vi "test Add Import Deploy.vi"(8 "error in":errorcluster, 11 "TestCase in":refnum<class "Examples.lvclass">) -> (0 "error out":errorcluster, 3 "TestCase out":refnum<class "Examples.lvclass">)   [LabVIEW 2024, in "Examples.lvclass"]
uses:
  Examples.lvclass
  C:/Program Files/National Instruments/LabVIEW 2024/vi.lib/NI/VeriStand Custom Device Testing Tools/VeriStandTestCase/VeriStandTestCase.lvclass
  Examples.lvclass/Examples.ctl
  7f6914e5-79d7-41a5-a6cd-be6651e4326d.vi
  <vilib>/addons/_JKI Toolkits/VI Tester/TestCase.llb/TestCase.lvclass
  C:/Program Files/National Instruments/LabVIEW 2024/vi.lib/addons/_JKI Toolkits/VI Tester/TestCase.llb/TestCase.lvclass
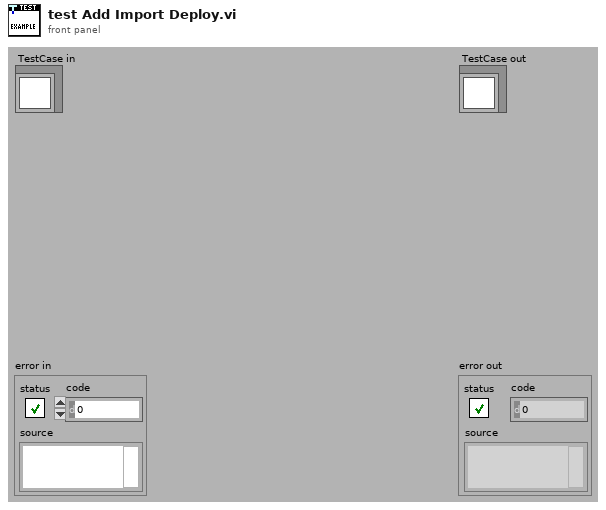
[diagram p1: front panel]
types:
  T1 = typedef "NI_VS Workspace ExecutionAPI.lvlib/WorkspaceAPI.ctl" = refnum<k24>
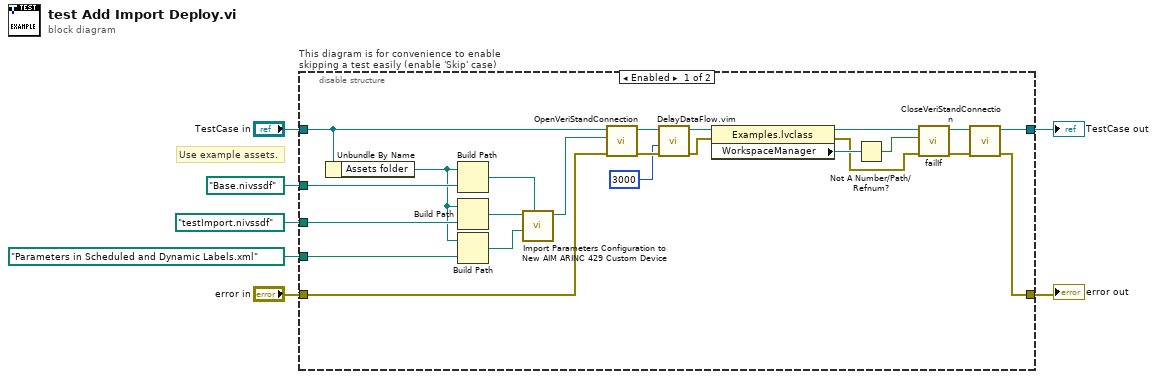
[diagram p0: block diagram]
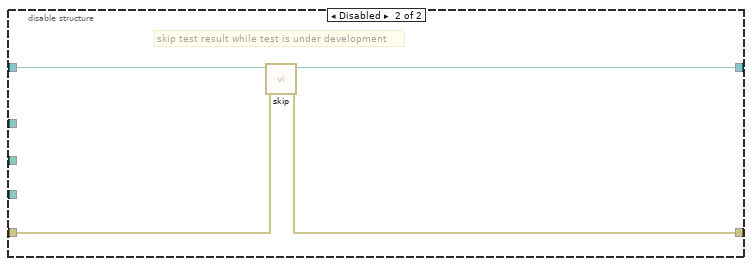
[diagram p2: hidden frame]
diagram:
  # "Use example assets."
  n1 = disable-structure "This diagram is for convenience to enable skipping a test easily (enable 'Skip' case)" shown="Enabled" {
    disable-tunnel: "TestCase in" -> [w16 w33]
    disable-tunnel: [w17 w31] -> w4
    disable-tunnel: [w18 w32] -> w6
    disable-tunnel: "error in" -> [w15 w30]
    disable-tunnel: path "Parameters in Scheduled and Dynamic Labels.xml" ("name or relative path") -> [w29 _]
    disable-tunnel: path "Base.nivssdf" ("name or relative path") -> [w13 _]
    disable-tunnel: path "testImport.nivssdf" ("name or relative path") -> [w12 _]
    frame Enabled {
      n2 = Unbundle By Name(w16) -> ("Assets folder"=w11:path)
      n3 = Build Path(base path=w11, name or relative path=w13) -> (appended path=w8:path)
      n4 = Build Path(base path=w11, name or relative path=w12) -> (appended path=w9:path)
      n5 = Build Path(base path=w11, name or relative path=w29) -> (appended path=w10:path)
      n6 = call "Import Parameters Configuration to New AIM ARINC 429 Custom Device.vi"("Base System Definition File"=w8, "Parameters Configuration File"=w10, "Output System Definition File"=w9) -> ("AIM ARINC 429 System Definition"=w14:path)  [unwired: 8 in]
      n7 = call-dynamic "OpenVeriStandConnection.vi"("error in (no error)"=w15, "System Definition File"=w14, "VeriStand Test Case in"=w16) -> ("error out"=w21:errorcluster, "VeriStand Test Case out"=w20:refnum<class "Examples.lvclass">)  [unwired: 6 in, 1 out]
      n8 = call "DelayDataFlow.vim"("value in"=w21, "milliseconds to wait"=u32 3000) -> ("value out"=w28:errorcluster)  [unwired: 2 in, 1 out]
      n9 = property class="Examples.lvclass"(reference=w20, error in=w28) -> (reference out=w27:refnum<class "Examples.lvclass">, error out=w22:errorcluster, "WorkspaceManager"=w24:T1)
      n10 = Not A Number/Path/Refnum?(number/path/refnum=w24) -> (NaN/Path/Refnum?=w23:bool)
      n11 = call-dynamic "failIf.vi"("error in (no error)"=w22, "fail"=w23, "TestCase in"=w27) -> ("error out"=w25:errorcluster, "TestCase out"=w26:refnum<class "Examples.lvclass">)  [unwired: 7 in]
      n12 = call-dynamic "CloseVeriStandConnection.vi"("error in (no error)"=w25, "VeriStand Test Case in"=w26) -> ("error out"=w18:errorcluster, "VeriStand Test Case out"=w17:refnum<class "Examples.lvclass">)  [unwired: 8 in]
    }
    frame Disabled {
      # "skip test result while test is under development"
      n13 = call <vilib>:"skip.vi"("error in (no error)"=w30, "TestCase in"=w33) -> ("error out"=w32:errorcluster, "TestCase out"=w31:refnum<class "Examples.lvclass">)  [unwired: 8 in]
    }
  }
  "error out" <- w6
  "TestCase out" <- w4
